vi "global counter.vi"() -> (3 "message ID":u8)   [LabVIEW 2013, in "Standard Engine Runtime.lvclass"]
uses:
  Standard Engine Runtime.lvclass
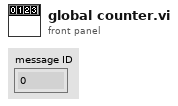
[diagram p1: front panel]
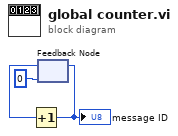
[diagram p0: block diagram]
diagram:
  n1 = feedback #1(u8 0) -> (w2:u8)
  n2 = Increment(x=w2) -> (x+1=w3:u8)
  "message ID" <- w3
  n3 = feedback-in #1(w3) -> ()
